vi "初始化默认值.vi"(8 "error in (no error)":errorcluster caption="错误输入（无错误）", 11 "段- 输入":refnum<class "段-.lvclass">) -> (0 "error out":errorcluster caption="错误输出", 3 "段- 输出":refnum<class "段-.lvclass">)   [LabVIEW 2017, in "项目开发助手.lvlib" / "模板-配置文件相关.lvlib" / "段-.lvclass"]
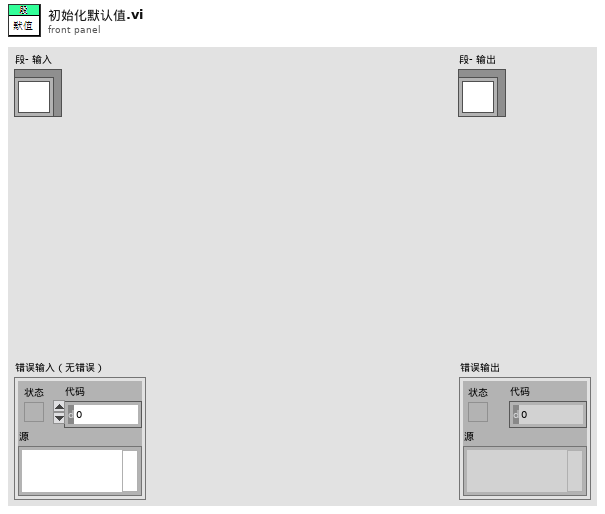
[diagram p1: front panel]
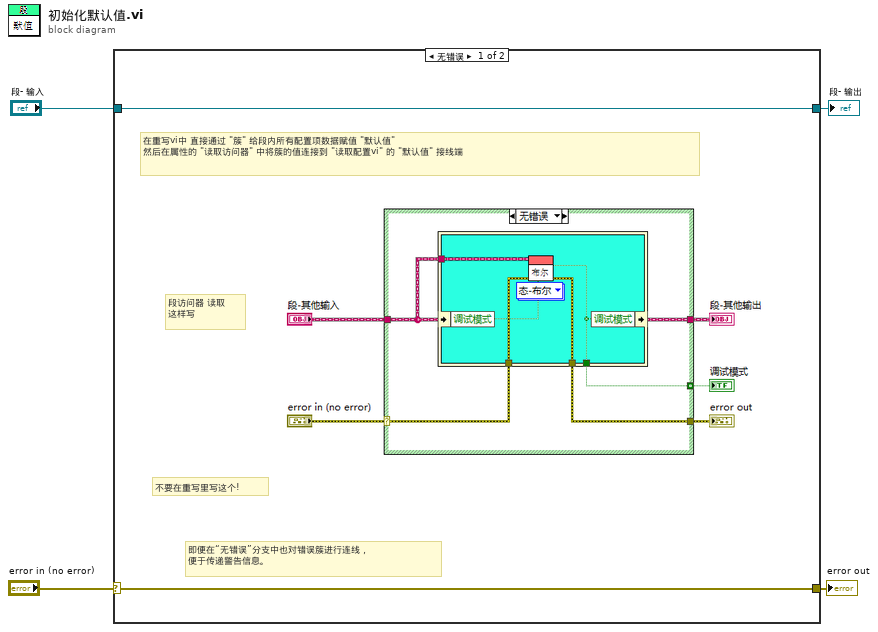
[diagram p0: block diagram]
diagram:
  n1 = case shown="无错误" "error in (no error)" {
    selector: "error in (no error)" -> [w5 w8]
    tunnel: [w5 w8] -> w3
    tunnel: [w6 w7] -> w1
    tunnel: "段- 输入" -> [w6 w7]
    frame No Error {
      # "不要在重写里写这个!"
      # "段访问器 读取\n这样写"
      # "在重写vi中 直接通过 \"簇\" 给段内所有配置项数据赋值 \"默认值\"\n然后在属性的 \"读取访问器\" 中将簇的值连接到 \"读取配置vi\" 的 \"默认值\" 接线端"
      # "即便在“无错误”分支中也对错误簇进行连线，\n便于传递警告信息。"
    }
    frame Error {
    }
  }
  "error out" <- w3
  "段- 输出" <- w1
